vi "Corece To Tiff Type.vi"(7 "Allowed Types":T2[](array[typedef]), 8 "error in (no error)":errorcluster, 10 "Variant Data type (optional)":T1, 11 "Variant":variant) -> (0 "error out":errorcluster, 2 "Actual Type":T2, 3 "Coerced Variant":variant)   [LabVIEW 2020, in "LV Tiff.lvlib"]
uses:
  LV Tiff.lvlib
  Tiff Data Type.ctl
  <vilib>/Utility/Data Type/Type Definitions/Data Type.ctl
  <vilib>/Utility/Data Type/NI_Data Type.lvlib
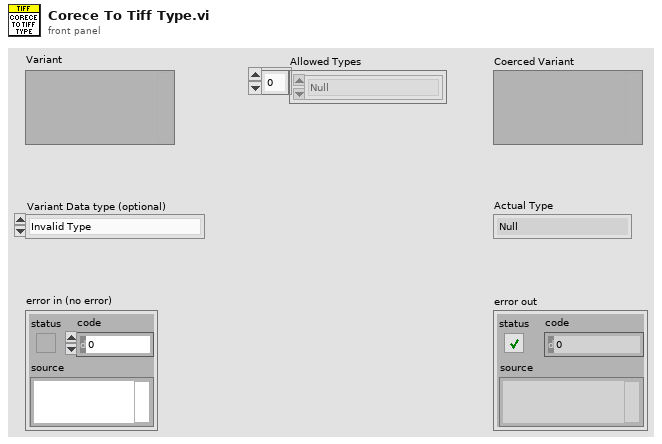
[diagram p1: front panel]
types:
  T1 = typedef "NI_Data Type.lvlib/Data Type.ctl" = enum8{"Invalid Type", "Void", "I8", "I16", "I32", "I64", "U8", "U16", "U32", "U64", "Single Float", "Double Float", "Extended Float", "Single Complex", "Double Complex", "Extended Complex", "Enum U8", "Enum U16", "Enum U32", "Enum U64", "Single Float With Unit", "Double Float With Unit", "Extended Float With Unit", "Single Complex with Unit", "Double Complex with Unit", "Extended Complex with Unit", "Boolean", "String", "Path", "Picture", "Tag", "Array", "Cluster", "Variant", "LV Variant", "Waveform", "Timestamp", "Digital Waveform", "Digital Data", "ExpressData", "Refnum", "External Data", "VI", "Poly VI", "LabVIEW Class Instance", "Fixed Point", "Set Collection", "Map Collection"}
  T2 = typedef "LV Tiff.lvlib/Tiff Data Type.ctl" = enum16{"Null", "BYTE", "ASCII", "SHORT", "LONG", "RATIONAL", "SBYTE", "UNDEFINE", "SSHORT", "SLONG", "SRATIONAL", "FLOAT", "DOUBLE"}
  T3 = enum16{"big-endian, network order", "native, host order", "little-endian"}
  T4 = cluster{"type string":i16[], "data string":string}
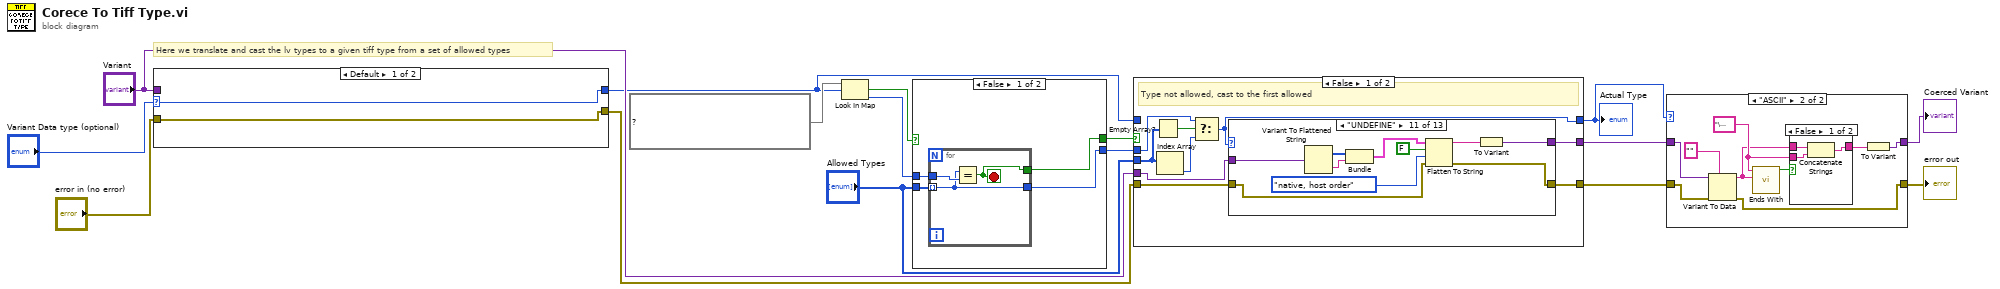
[diagram p0: block diagram]
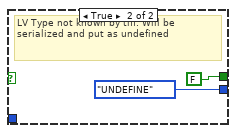
[diagram p2: hidden frame]
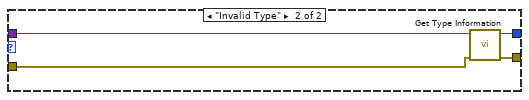
[diagram p3: hidden frame]
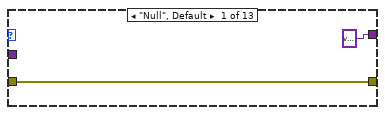
[diagram p6: hidden frame]
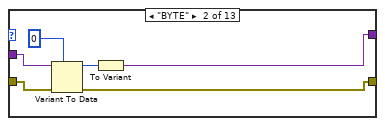
[diagram p7: hidden frame]
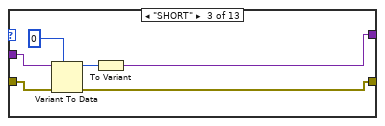
[diagram p8: hidden frame]
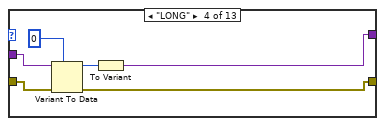
[diagram p9: hidden frame]
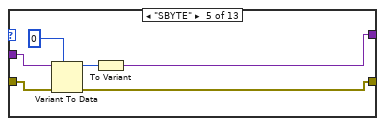
[diagram p10: hidden frame]
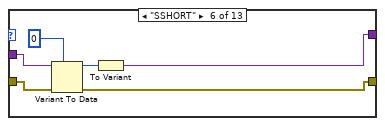
[diagram p11: hidden frame]
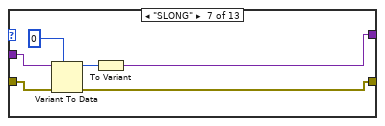
[diagram p12: hidden frame]
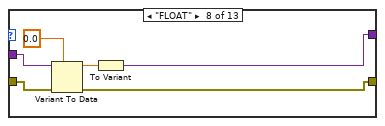
[diagram p13: hidden frame]
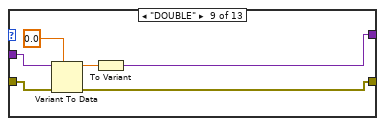
[diagram p14: hidden frame]
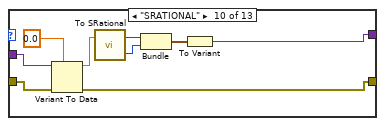
[diagram p15: hidden frame]
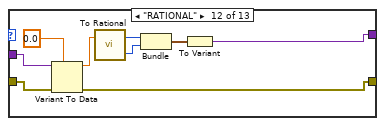
[diagram p16: hidden frame]
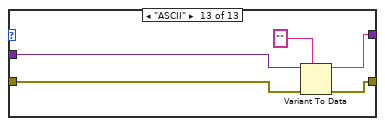
[diagram p17: hidden frame]
diagram:
  # "Here we translate and cast the lv types to a given tiff type from a set of allowed types"
  n1 = case shown="Default" "Variant Data type (optional)" {
    selector: "Variant Data type (optional)" -> [w17 _]
    tunnel: "Variant" -> [_ w22]
    tunnel: [w17 w21] -> w11
    tunnel: [w18 w20] -> w10
    tunnel: "error in (no error)" -> [w18 w19]
    frame Default {
    }
    frame "Invalid Type" {
      n2 = call <vilib>:"Get Type Information.vi"("error in (no error)"=w19, "variant"=w22) -> ("error out"=w20:errorcluster, "type"=w21:T1)  [unwired: 5 in, 3 out]
    }
  }
  n3 = Look In Map(map=map{T1, T2} {enum."Invalid Type"=enum."UNDEFINE", enum."I8"=enum."SBYTE", enum."I16"=enum."SSHORT", enum."I32"=enum."SLONG", enum."U8"=enum."BYTE", enum."U16"=enum."SHORT", enum."U32"=enum."LONG", enum."Single Float"=enum."FLOAT", enum."Double Float"=enum."DOUBLE", enum."String"=enum."ASCII"}, key=w11) -> (key not found?=w1:bool, value=w15:T2)  [unwired: 1 in]
  n4 = case shown="False" w1 {
    tunnel: w15 -> [w26 _]
    tunnel: [w25 FALSE] -> w14
    tunnel: "Allowed Types" -> [w24 _]
    tunnel: [w23 Tiff_Data_Type."UNDEFINE" ("DataType")] -> w8
    frame False {
      n5 = for {
        tunnel: w24 -> [w27] mode=indexing
        tunnel: w26 -> [w29]
        tunnel: [w28] -> w25
        tunnel: [w27] -> w23
        stop <- w28 stop-if-true
        n6 = Equal?(x=w27, y=w29) -> (x = y?=w28:bool)
      }
    }
    frame True {
      # "LV Type not known by tiff. Will be serialized and put as undefined"
    }
  }
  n7 = case shown="False" w14 {
    tunnel: "Variant" -> [w40 w126]
    tunnel: [w39 w126] -> w6
    tunnel: "Allowed Types" -> [w35 _]
    tunnel: w11 -> [_ _]
    tunnel: w10 -> [w38 w125]
    tunnel: [w37 w125] -> w4
    tunnel: [w32 w124] -> w7
    tunnel: w8 -> [w33 w124]
    frame False {
      # "Type not allowed, cast to the first allowed"
      n8 = Empty Array?(array=w35) -> (empty?=w34:bool)
      n9 = Index Array(array=w35) -> (element=w36:T2)  [unwired: 1 in]
      n10 = Select(t=w33, s=w34, f=w36) -> (s? t:f=w32:T2)
      n11 = case shown="\"UNDEFINE\"" w32 {
        tunnel: w40 -> [_ w48 w54 w60 w66 w72 w78 w84 w90 w99 w108 w118 w123]
        tunnel: [variant ("Variant") w45 w51 w57 w63 w69 w75 w81 w87 w97 w109 w116 w119] -> w39
        tunnel: w38 -> [w41 w44 w50 w56 w62 w68 w74 w80 w86 w96 w103 w115 w121]
        tunnel: [w41 w43 w49 w55 w61 w67 w73 w79 w85 w95 w102 w114 w120] -> w37
        frame "Null", Default {
        }
        frame "BYTE" {
          n12 = Variant To Data(error in=w44, type=u8 0, Variant=w48) -> (data=w46:u8, error out=w43:errorcluster)
          n13 = To Variant(anything=w46) -> (Variant=w45:variant)
        }
        frame "SHORT" {
          n14 = Variant To Data(error in=w50, type=u16 0, Variant=w54) -> (data=w52:u16, error out=w49:errorcluster)
          n15 = To Variant(anything=w52) -> (Variant=w51:variant)
        }
        frame "LONG" {
          n16 = Variant To Data(error in=w56, type=u32 0, Variant=w60) -> (data=w58:u32, error out=w55:errorcluster)
          n17 = To Variant(anything=w58) -> (Variant=w57:variant)
        }
        frame "SBYTE" {
          n18 = Variant To Data(error in=w62, type=i8 0, Variant=w66) -> (data=w64:i8, error out=w61:errorcluster)
          n19 = To Variant(anything=w64) -> (Variant=w63:variant)
        }
        frame "SSHORT" {
          n20 = Variant To Data(error in=w68, type=i16 0, Variant=w72) -> (data=w70:i16, error out=w67:errorcluster)
          n21 = To Variant(anything=w70) -> (Variant=w69:variant)
        }
        frame "SLONG" {
          n22 = Variant To Data(error in=w74, type=0, Variant=w78) -> (data=w76:i32, error out=w73:errorcluster)
          n23 = To Variant(anything=w76) -> (Variant=w75:variant)
        }
        frame "FLOAT" {
          n24 = Variant To Data(error in=w80, type=sgl 0.0, Variant=w84) -> (data=w82:sgl, error out=w79:errorcluster)
          n25 = To Variant(anything=w82) -> (Variant=w81:variant)
        }
        frame "DOUBLE" {
          n26 = Variant To Data(error in=w86, type=0.0, Variant=w90) -> (data=w88:dbl, error out=w85:errorcluster)
          n27 = To Variant(anything=w88) -> (Variant=w87:variant)
        }
        frame "SRATIONAL" {
          n28 = Variant To Data(error in=w96, type=0.0, Variant=w99) -> (data=w94:dbl, error out=w95:errorcluster)
          n29 = call "To SRational.vi"("Number"=w94) -> ("Denominator"=w91:i32, "Numerator"=w92:i32)  [unwired: 1 in]
          n30 = Bundle("Numerator"=w92, "Denominator"=w91) -> (w93:cluster{"Numerator":i32, "Denominator":i32})  [unwired: 1 in]
          n31 = To Variant(anything=w93) -> (Variant=w97:variant)
        }
        frame "UNDEFINE" {
          n32 = Variant To Flattened String(Variant=w108) -> (data string=w106:string, 1:w107:i16[])
          n33 = Bundle("type string"=w107, "data string"=w106) -> (w105:T4)  [unwired: 1 in]
          n34 = Flatten To String(anything=w105, prepend array or string size? (T)=FALSE, byte order (0:big-endian, network order)=T3."native, host order", error in (no error)=w103) -> (data string=w101:string, error out=w102:errorcluster)  [unwired: 1 out]
          n35 = To Variant(anything=w101) -> (Variant=w109:variant)
        }
        frame "RATIONAL" {
          n36 = Variant To Data(error in=w115, type=0.0, Variant=w118) -> (data=w113:dbl, error out=w114:errorcluster)
          n37 = call "To Rational.vi"("Number"=w113) -> ("Divider"=w111:u32, "Numerator"=w112:u32)  [unwired: 1 in]
          n38 = Bundle("Numerator"=w112, "Divider"=w111) -> (w110:cluster{"Numerator":u32, "Divider":u32})  [unwired: 1 in]
          n39 = To Variant(anything=w110) -> (Variant=w116:variant)
        }
        frame "ASCII" {
          n40 = Variant To Data(error in=w121, type="", Variant=w123) -> (data=w119:string, error out=w120:errorcluster)
        }
      }
    }
    frame True {
      # "This type is allowed, so no cast needed"
    }
  }
  "Actual Type" <- w7
  n41 = case shown="\"ASCII\"" w7 {
    tunnel: w6 -> [w127 w134]
    tunnel: [w127 w132] -> w5
    tunnel: w4 -> [w128 w130]
    tunnel: [w128 w129] -> w3
    frame Default {
    }
    frame "ASCII" {
      w135 = "\u0000" ("Suffix")
      n42 = Variant To Data(error in=w130, type="", Variant=w134) -> (data=w131:string, error out=w129:errorcluster)
      n43 = call "Ends With.vi"("String"=w131, "Suffix"=w135) -> ("Ended with"=w137:bool)  [unwired: 8 in, 1 out]
      n44 = case shown="False" w137 {
        tunnel: [w139 w141] -> w136
        tunnel: w131 -> [w140 w141]
        tunnel: w135 -> [w138 _]
        frame False {
          n45 = Concatenate Strings(w140, w138) -> (w139:string)
        }
        frame True {
        }
      }
      n46 = To Variant(anything=w136) -> (Variant=w132:variant)
    }
  }
  "Coerced Variant" <- w5
  "error out" <- w3
